vi "Validate Response.vi"(8 "error in (no error)":errorcluster, 10 "Response Data":T1, 11 "Text based Communications Test in":refnum<class "Text based Communications Test.lvclass">) -> (0 "error out":errorcluster, 3 "Text based Communications Test out":refnum<class "Text based Communications Test.lvclass">)   [LabVIEW 2017, in "Text based Communications Test.lvlib" / "Text based Communications Test.lvclass"]
uses:
  Text based Communications Test.lvclass
  File Data Format.ctl
  Text based Communications Test.lvclass/Text based Communications Test.ctl
  Text based Communications Test.lvlib
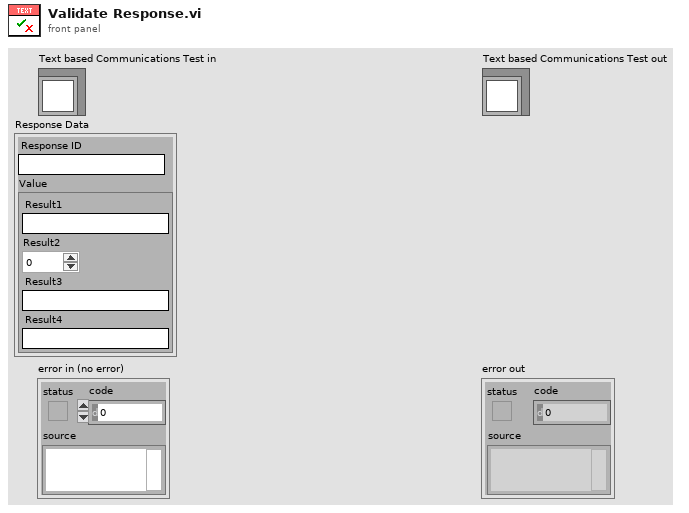
[diagram p1: front panel]
types:
  T1 = typedef "Text based Communications Test.lvlib/File Data Format.ctl" = cluster{"Response ID":string, "Value":cluster{"Result1":string, "Result2":dbl, "Result3":string, "Result4":string}}
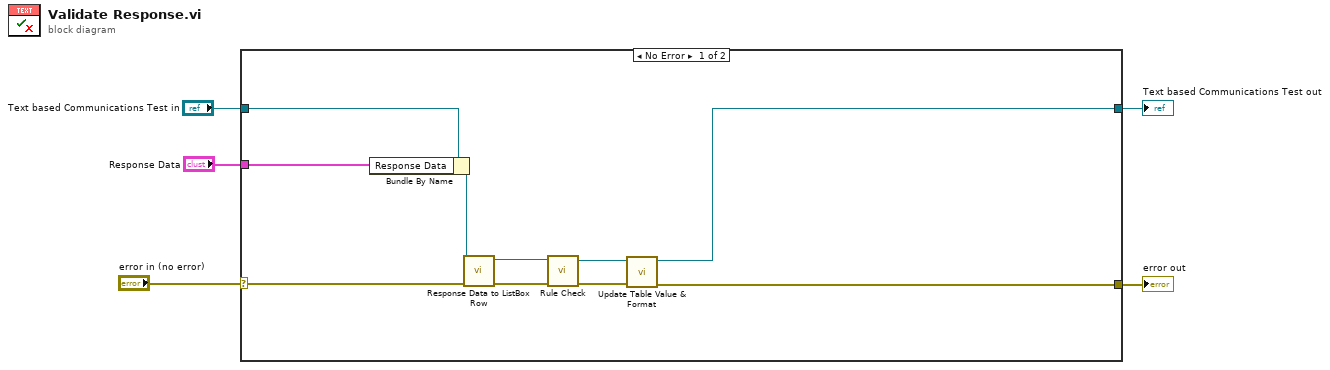
[diagram p0: block diagram]
diagram:
  n1 = case shown="No Error" "error in (no error)" {
    selector: "error in (no error)" -> [w12 w17]
    tunnel: [w9 w17] -> w4
    tunnel: [w8 w16] -> w2
    tunnel: "Text based Communications Test in" -> [w15 w16]
    tunnel: "Response Data" -> [w6 _]
    frame No Error {
      n2 = Bundle By Name(cluster=w15, "Response Data"=w6) -> (w7:refnum<class "Text based Communications Test.lvclass">)
      n3 = call "Response Data to ListBox Row.vi"("error in (no error)"=w12, "Text based Communications Test in"=w7) -> ("error out"=w13:errorcluster, "Text based Communications Test out"=w14:refnum<class "Text based Communications Test.lvclass">)  [unwired: 8 in]
      n4 = call "Rule Check.vi"("error in (no error)"=w13, "Text based Communications Test in"=w14) -> ("error out"=w11:errorcluster, "Text based Communications Test out"=w10:refnum<class "Text based Communications Test.lvclass">)  [unwired: 8 in]
      n5 = call "Update Table Value & Format.vi"("error in (no error)"=w11, "Text based Communications Test in"=w10) -> ("error out"=w9:errorcluster, "Text based Communications Test out"=w8:refnum<class "Text based Communications Test.lvclass">)  [unwired: 8 in]
    }
    frame Error {
    }
  }
  "error out" <- w4
  "Text based Communications Test out" <- w2
